vi "PSF_Estimation.vi"(7 "xnorm_um_scaling":dbl, 8 "error in (no error)":errorcluster, 10 "filter_size":dbl, 11 "detection_threshold":dbl=0.8 format="%#_13g") -> (0 "error out":errorcluster)   [LabVIEW 2020]
uses:
  Global Variables/General Globals.vi
  Global Variables/gl_UI Ctrl Refs.vi
panel:
  out "result":dbl
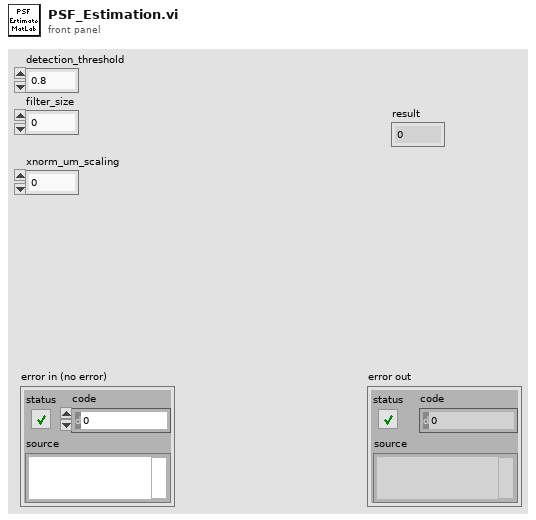
[diagram p1: front panel]
types:
  T1 = typedef "UI ctrl refs cluster.ctl" = cluster{"Top level VI path":path, "Top level VI ref":refnum<vi>, "User menu ref":refnum<k9>, "Sub Panel control":refnum<vi>, "Imaging Param Tab":refnum<vi>, "Occurrence-Start drivers":refnum<k4>, "Occurrence-Speed logging initialised":refnum<k4>, "Occurrence-XYZ stage initialised":refnum<k4>, "Exit button":refnum<vi>, "Status ind":refnum<vi>, "Set as origin":refnum<vi>, "Speed Logging":refnum<vi>, "Time Lapse":refnum<vi>, "Live Imaging":refnum<vi>, "AOL Z Stack":refnum<vi>, "Motor Z Stack":refnum<vi>, "Funct Acq button":refnum<vi>, "Hard Shutter":refnum<vi>, "Virtual Shutter":refnum<vi>, "Laser Power":refnum<vi>, "AOL Mode":refnum<vi>, "Frame Size":refnum<vi>, "Field of View":refnum<vi>, "Dwell Time":refnum<vi>, "Zoom":refnum<vi>, "AOL Z":refnum<vi>, "Objective":refnum<vi>, "Axis":refnum<vi>, "Paths & Names":refnum<vi>, "Experiment folder path (ind.)":refnum<vi>, "Last State (Ind.)":refnum<vi>, "Averages":refnum<vi>, "Angle (degrees)":refnum<vi>, "X centre":refnum<vi>, "Y centre":refnum<vi>, "Plane Mode":refnum<vi>, "# Planes":refnum<vi>, "Z Start":refnum<vi>, "Z Stop":refnum<vi>, "Z Step":refnum<vi>, "PMT 1":refnum<vi>, "PMT 2":refnum<vi>, "Stage XYZ Position":refnum<vi>, "Pockels@Z Start":refnum<vi>, "Pockels@Z Stop":refnum<vi>, "Obtain Z Start":refnum<vi>, "Obtain Z Stop":refnum<vi>, "Live stim.trig.period":refnum<vi>, "Live stim.trig.enable":refnum<vi>, "Movement Correction":refnum<vi>, "Load Reference Image":refnum<vi>, "XY Stage Move":refnum<vi>, "MovCor Cluster":refnum<vi>, "RefDAQParam":refnum<vi>, "Funct. Acq. Pockels Modulation":refnum<vi>, "Ref Laser Power":refnum<vi>, "Enable Video Recording":refnum<vi>, "Video Record-Live Imaging":refnum<vi>, "Video Record-Funct acq":refnum<vi>, "Reference Source":refnum<vi>, "AOL Z-stack Chirps Ready (ind)":refnum<vi>, "Target time between mov.cor. ref triggers (ms)":refnum<vi>, "Funct. Acq. Ref frame save":refnum<vi>, "Tracking button":refnum<vi>, "Show ref plots window":refnum<vi>, "Center freq ind (nm)":refnum<vi>, "Pickup mode (ind)":refnum<vi>, "Logging queue (ind)":refnum<vi>, "Back aperture power (ind.)":refnum<vi>, "Power after objective (ind.)":refnum<vi>, "Switch user":refnum<vi>, "Ls1 Conn. Status":refnum<vi>, "Ls1Tuning Status":refnum<vi>, "Ls1 Faults":refnum<vi>, "Ls1 Connection":refnum<vi>, "Ls1 Mode":refnum<vi>, "Ls1 POWER [mW]":refnum<vi>, "Ls1Shutter":refnum<vi>, "Ls1 Wavelength":refnum<vi>, "Ls1 Note":refnum<vi>, "Ls1 Confirm Wav":refnum<vi>, "Ls1 PreChrp Prism1":refnum<vi>, "Ls1 PreChrp Prism2":refnum<vi>, "Ls1 wav top Ind":refnum<vi>, "Ls1 power top Ind":refnum<vi>, "Ls1 Pump peak Hold":refnum<vi>, "Ls1 Status Ind":refnum<vi>, "Ls1 wav cancel":refnum<vi>, "Experiment Type":refnum<vi>, "Biology Information":refnum<vi>}
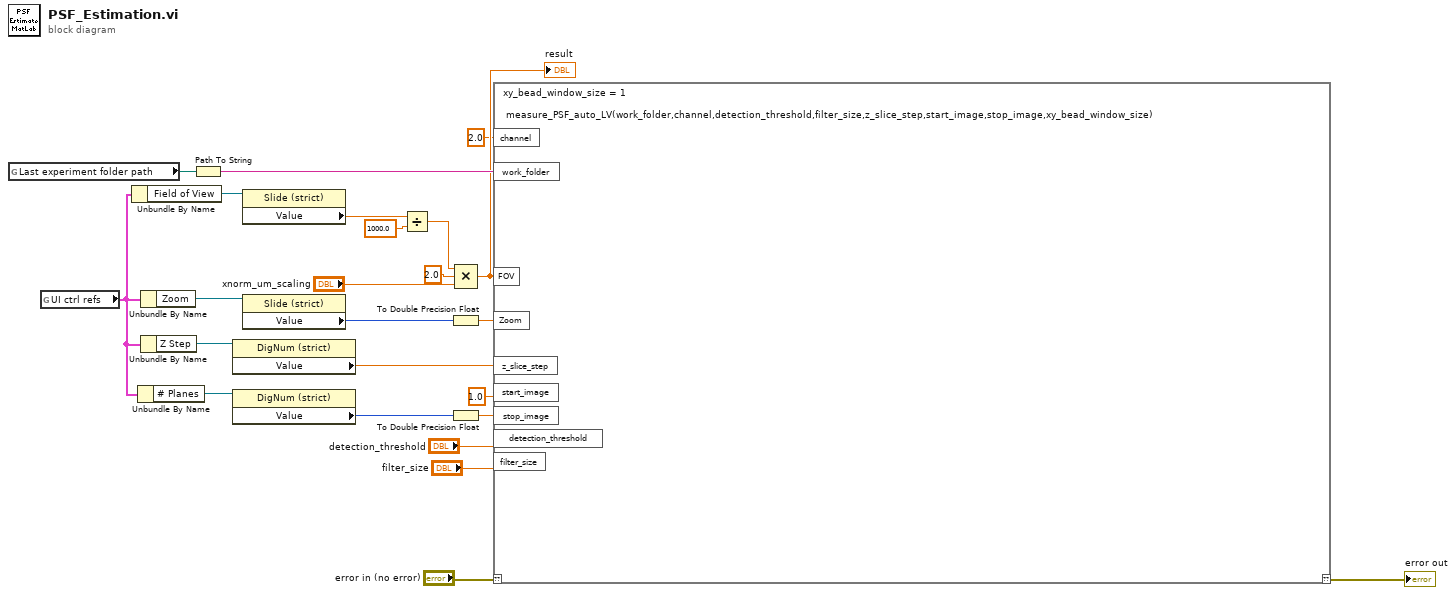
[diagram p0: block diagram]
diagram:
  n1 = global read "General Globals.vi" "Last experiment folder path"() -> (w19:path)
  n2 = global read "gl_UI Ctrl Refs.vi" "UI ctrl refs"() -> (w20:T1)
  n3 = Unbundle By Name(w20) -> ("Field of View"=w24:refnum<vi>)
  n4 = Unbundle By Name(w20) -> ("# Planes"=w21:refnum<vi>)
  n5 = Unbundle By Name(w20) -> ("Zoom"=w23:refnum<vi>)
  n6 = Unbundle By Name(w20) -> ("Z Step"=w22:refnum<vi>)
  n7 = Path To String(path=w19) -> (string=w18:string)
  n8 = property class="DigNum (strict)"(reference=w22) -> ("Value"=w15:dbl)  [unwired: 1 in, 2 out]
  n9 = property class="DigNum (strict)"(reference=w21) -> ("Value"=w14:u16)  [unwired: 1 in, 2 out]
  n10 = property class="Slide (strict)"(reference=w24) -> ("Value"=w8:sgl)  [unwired: 1 in, 2 out]
  n11 = property class="Slide (strict)"(reference=w23) -> ("Value"=w17:i8)  [unwired: 1 in, 2 out]
  n12 = Divide(x=w8, y=1000.0) -> (x/y=w12:dbl)
  n13 = To Double Precision Float(number=w17) -> (double precision float=w16:dbl)
  n14 = To Double Precision Float(number=w14) -> (double precision float=w13:dbl)
  n15 = Compound Arithmetic op=MULTIPLY(w12, 2.0 ("value"), "xnorm_um_scaling") -> (w7:dbl)
  "result" <- w7
  n16 = script code="xy_bead_window_size = 1\n\n measure_PSF_auto_LV(work_folder,channel,detection_threshold,filter_size,z_slice_step,start_image,stop_image,xy_bead_window_size)"("??"="error in (no error)", "work_folder"=w18, "FOV"=w7, "Zoom"=w16, "z_slice_step"=w15, "stop_image"=w13, "start_image"=1.0 ("Real"), "detection_threshold"="detection_threshold", "filter_size"="filter_size", "channel"=2.0 ("Real")) -> ("??"=→"error out":errorcluster)
